vi "Analysis MASTER.vi"(8 "Error In":errorcluster) -> (0 "Error Out":errorcluster)   [LabVIEW 2019, in "MainVIs.lvlib"]
uses:
  MainVIs.lvlib
  Analysis Support/Controls/Select Analysis.ctl
  Analysis Support/Controls/Master Analysis States.ctl
  AnalysisSupport.lvlib
panel:
  out "F0 Array (Mech)":dbl[](array[numeric])
  out "F0 Array (Labial)":dbl[](array[numeric])
  out "SPL Array (Mech)":dbl[](array[numeric])
  out "SPL Array (Labial)":dbl[](array[numeric])
  out "MFR (Labial)":dbl format="%0.3f"
  out "MFR (Mech)":dbl format="%0.3f"
  out "Start Flow (INC)":dbl format="%0.3f"
  out "End Flow (INC)":dbl format="%0.3f"
  out "PTP (INC)":dbl
  out "SPL (INC)":dbl format="%0.3f"
  out "SGP (INC)":dbl
  out "Resistance (INC)":dbl
  out "Pressure (Redirector)":dbl
  out "Filename Out":path
  out "Most Recent File Called":string
  out "SGP Array (Mech)":dbl[](array[numeric])
  out "PTP Array (Mech)":dbl[](array[numeric])
  out "Pressure Array (Labial)":dbl[](array[numeric])
  in  "Begin":bool
  out "Message":string
  in  "Analysis Type":T1 items=["Labial Interruption", "Mechanical Interruption", "Incomplete Interruption", "Airflow Redirection "]
  in  "Exit":bool
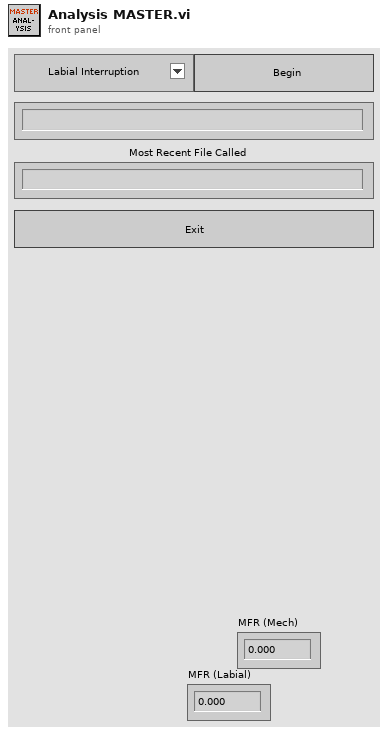
[diagram p1: front panel]
types:
  T1 = typedef "AnalysisSupport.lvlib/Select Analysis.ctl" = u16
  T2 = typedef "AnalysisSupport.lvlib/Master Analysis States.ctl" = enum16{"Initialize", "Wait to Start", "Analyze", "Save", "Timeout", "Exit"}
  T3 = enum16{"Left Button", "Center Button", "Right Button", "Window Close"}
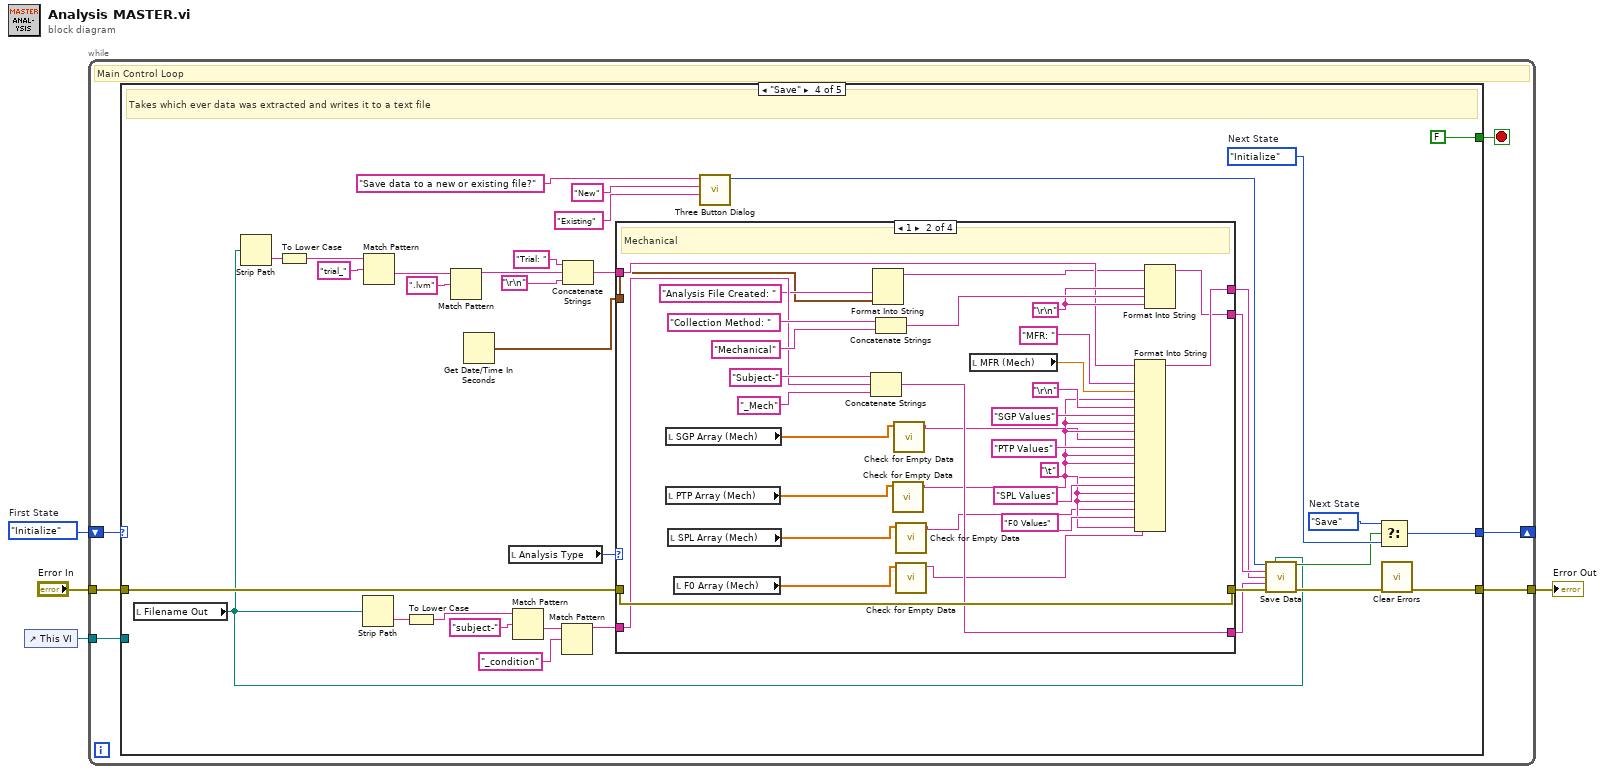
[diagram p0: block diagram]
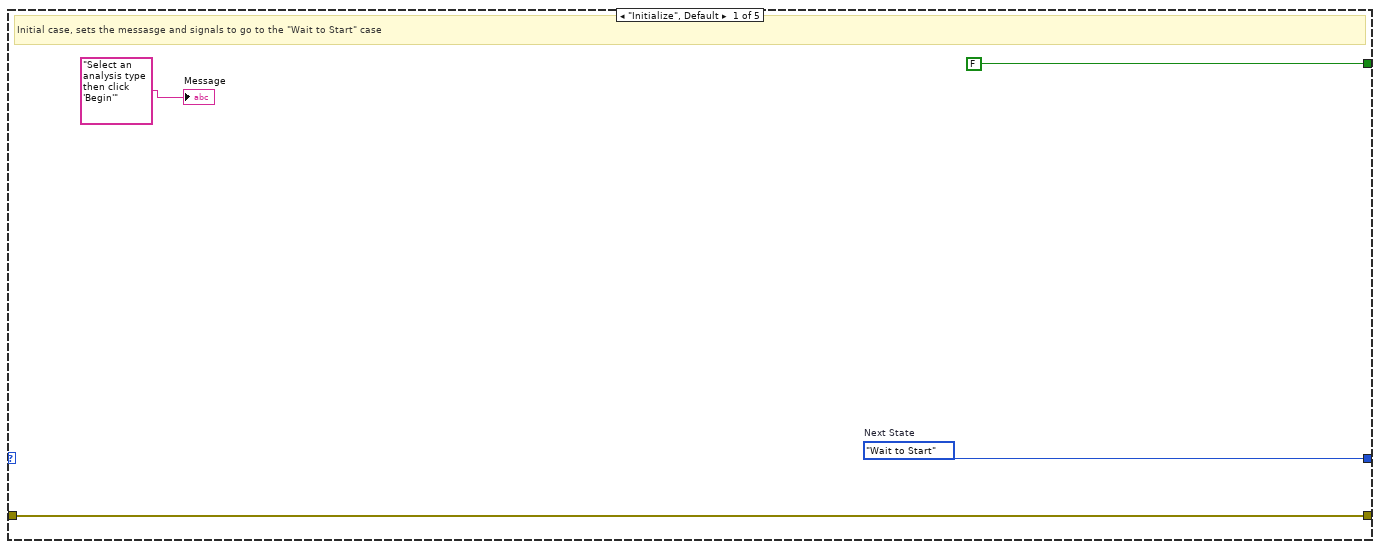
[diagram p2: hidden frame]
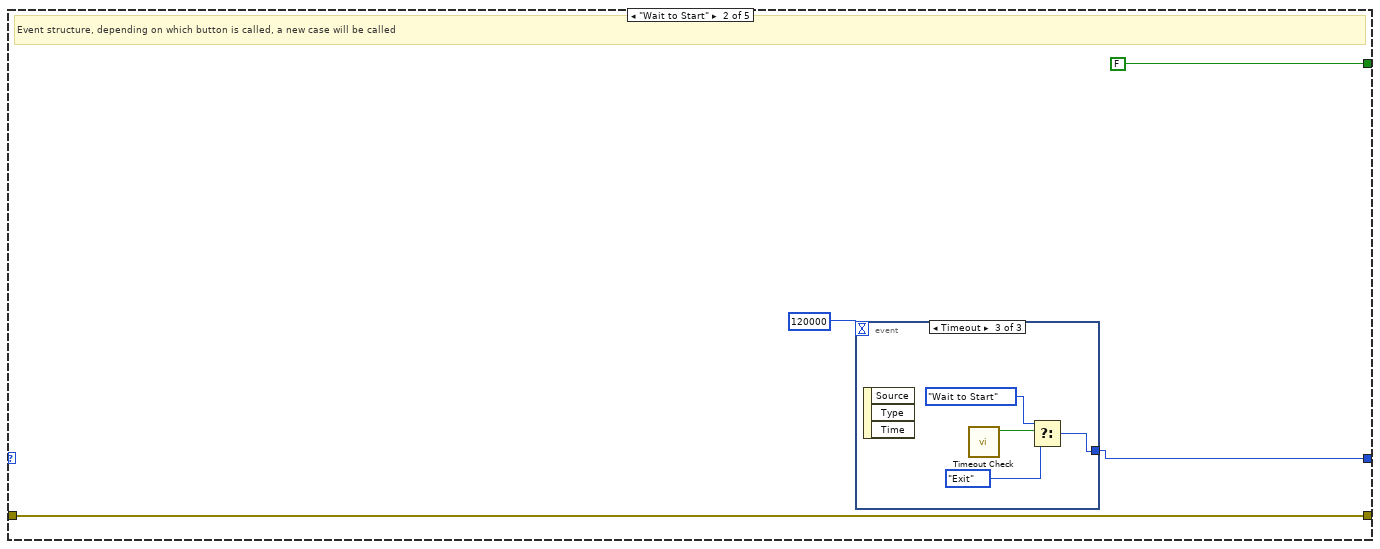
[diagram p3: hidden frame]
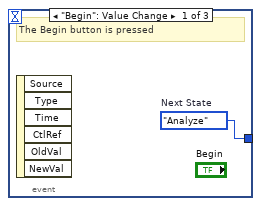
[diagram p4: hidden frame]
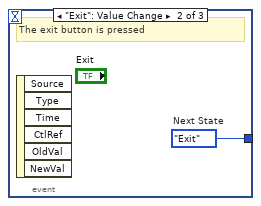
[diagram p5: hidden frame]
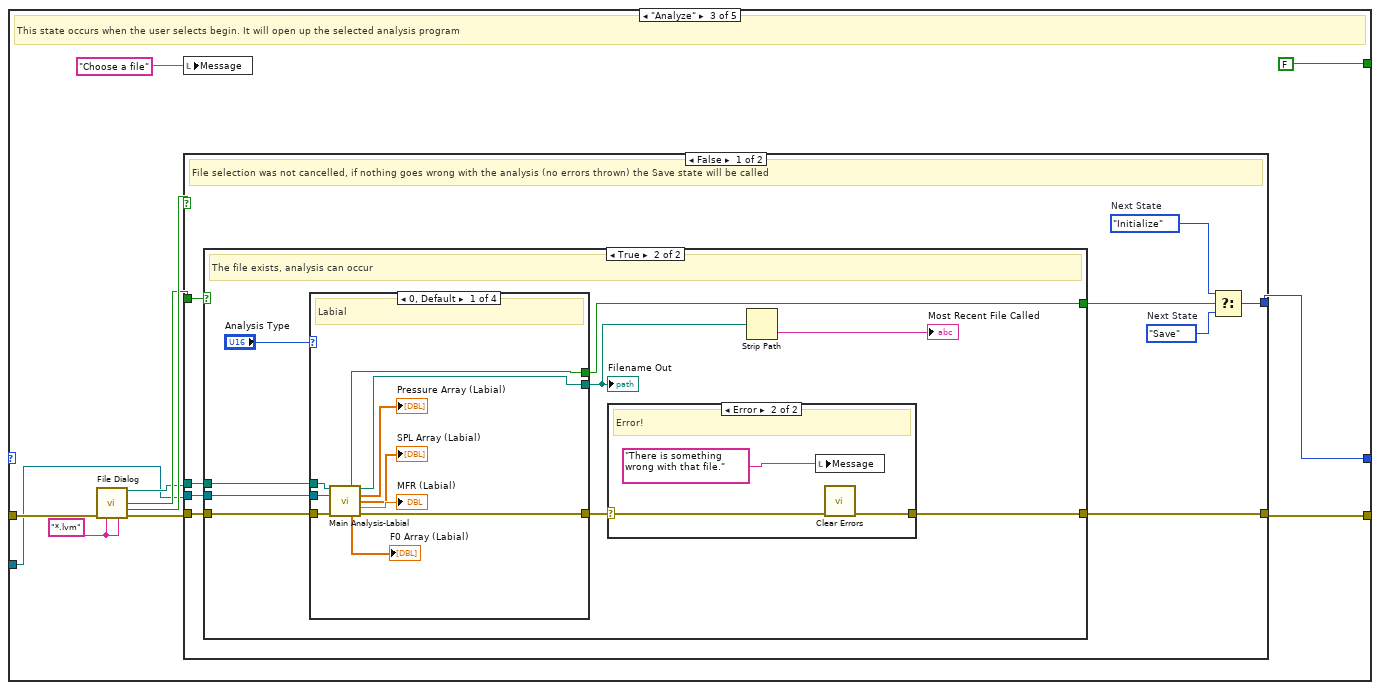
[diagram p6: hidden frame]
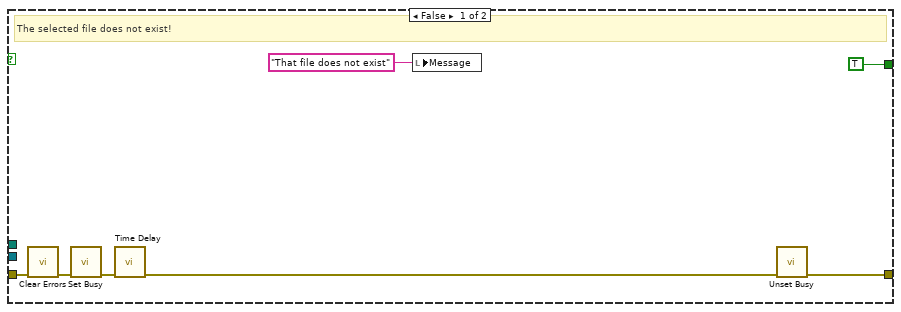
[diagram p7: hidden frame]
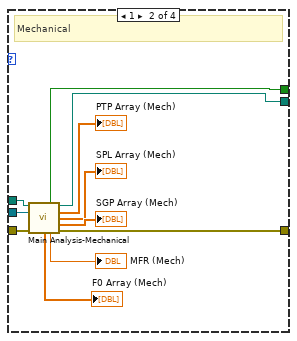
[diagram p9: hidden frame]
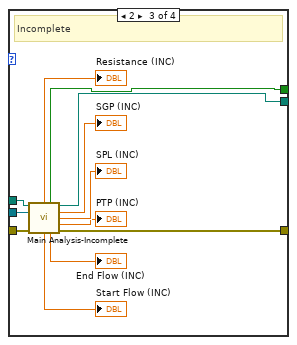
[diagram p10: hidden frame]
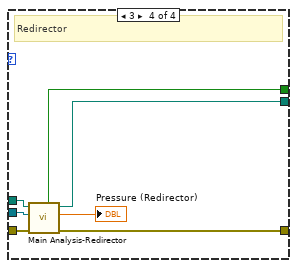
[diagram p11: hidden frame]
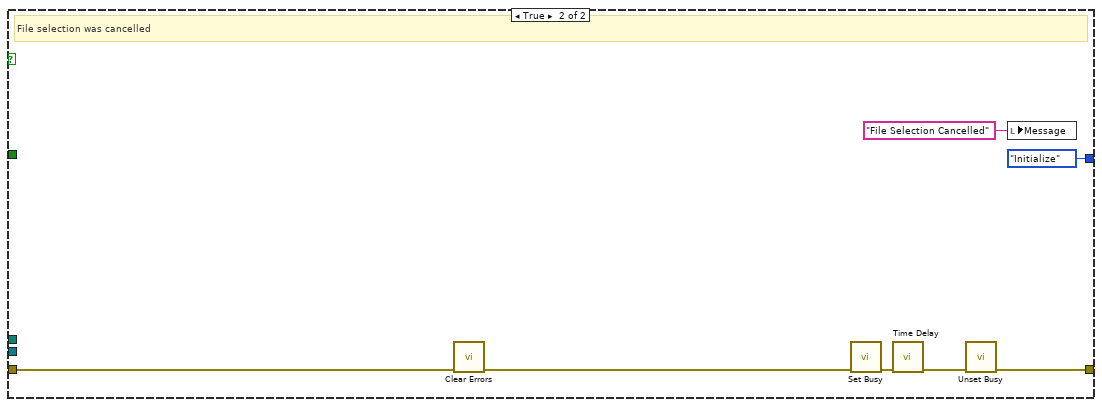
[diagram p12: hidden frame]
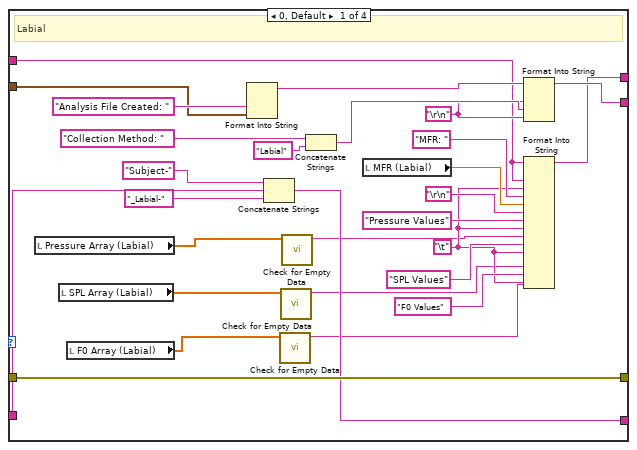
[diagram p13: hidden frame]
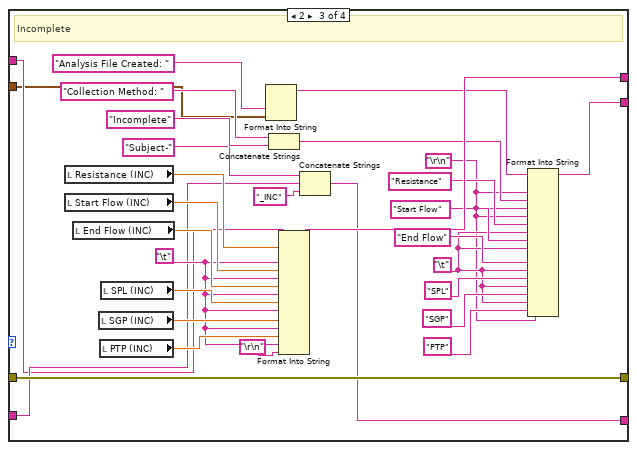
[diagram p14: hidden frame]
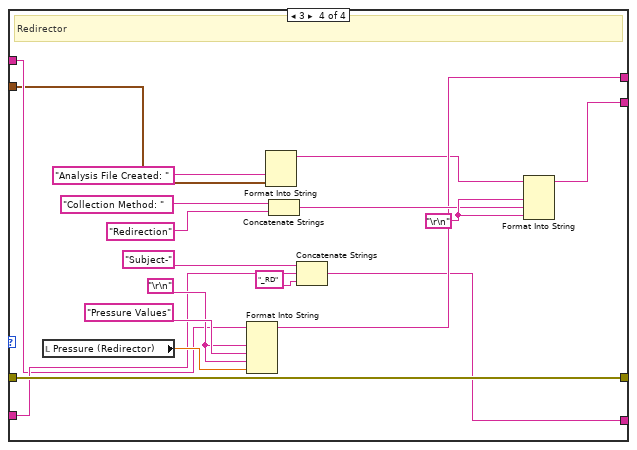
[diagram p15: hidden frame]
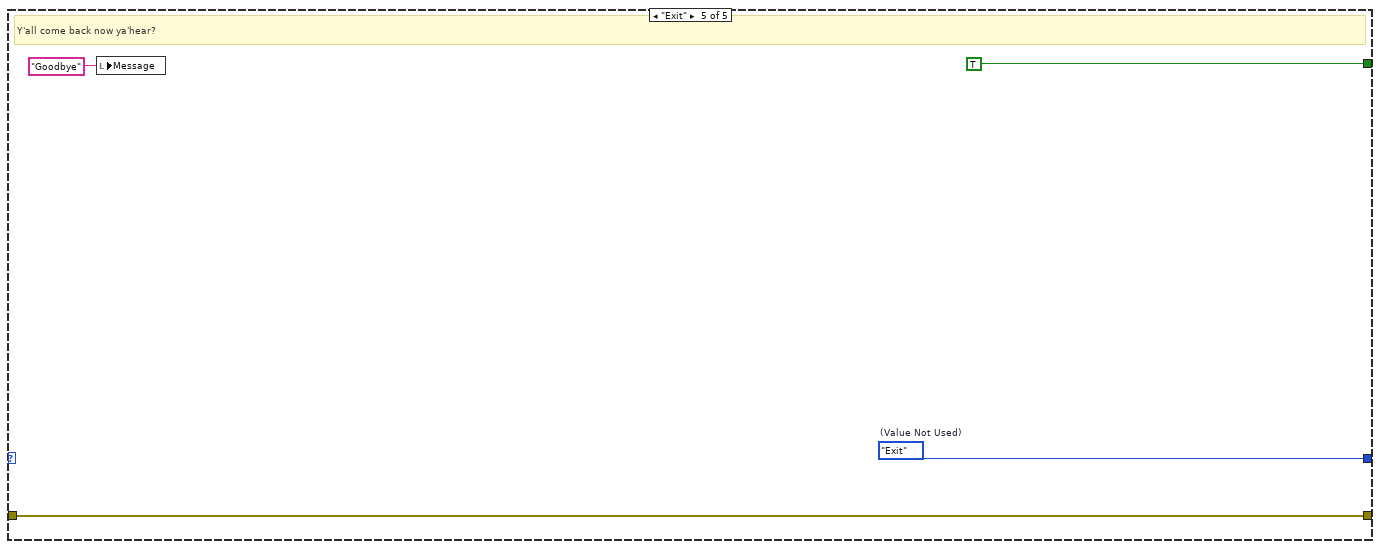
[diagram p16: hidden frame]
diagram:
  w4 = Master_Analysis_States."Initialize"  # First State
  n1 = control-ref of="This VI"() -> (w1:refnum<vi>)
  n2 = while {
    shift-right: [w8] -> _
    shift-left: w4 -> [w10]
    tunnel: "Error In" -> [w7]
    tunnel: [w6] -> w2
    tunnel: w1 -> [w5]
    stop <- w9 stop-if-true
    # "Main Control Loop"
    n3 = case shown="\"Save\"" w10 {
      tunnel: [FALSE FALSE FALSE FALSE TRUE] -> w9
      tunnel: [w12 w18 w26 w122 w255] -> w8
      tunnel: w7 -> [w11 w16 w33 w137 w253]
      tunnel: [w11 w16 w31 w144 w253] -> w6
      tunnel: w5 -> [_ _ w27 _ _]
      frame "Initialize", Default {
        w12 = Master_Analysis_States."Wait to Start"  # Next State
        # "Initial case, sets the messasge and signals to go to the \"Wait to Start\" case"
        "Message" <- "Select an analysis type then click 'Begin'" ("Message")
      }
      frame "Wait to Start" {
        # "Event structure, depending on which button is called, a new case will be called"
        n4 = event shown="[2] Timeout" {
          selector: _ -> [_ _ _]
          dyn-events: _ -> [_ _ _]
          timeout: 120000 -> [_ _ _]
          tunnel: [w19 w20 w21] -> w18
          event "Begin": Value Change {
            w19 = Master_Analysis_States."Analyze"  # Next State
            # "The Begin button is pressed"
            n5 = event-data() -> ()  [unwired: 1 in, 6 out]
          }
          event "Exit": Value Change {
            w20 = Master_Analysis_States."Exit"  # Next State
            # "The exit button is pressed"
            n6 = event-data() -> ()  [unwired: 1 in, 6 out]
          }
          event Timeout {
            n7 = event-data() -> ()  [unwired: 1 in, 3 out]
            n8 = call "Timeout Check.vi"() -> ("Still there?"=w24:bool)  [unwired: 10 in, 1 out]
            n9 = Select(t=Master_Analysis_States."Wait to Start" ("Next State"), s=w24, f=Master_Analysis_States."Exit") -> (s? t:f=w21:T2)
          }
        }
      }
      frame "Analyze" {
        w34 = "*.lvm" ("pattern (all files)")
        # "This state occurs when the user selects begin. It will open up the selected analysis program"
        n10 = call "File Dialog"("error in"=w33, "pattern (all files)"=w34, "pattern label"=w34) -> ("selected path"=w28:path, "exists"=w29:bool, "cancelled"=w30:bool, "error out"=w32:errorcluster)  [unwired: 9 in]
        n11 = local write "Message"("Choose a file" ("Message")) -> ()
        n12 = case shown="False" w30 {
          tunnel: w32 -> [w40 w108]
          tunnel: [w37 w107] -> w31
          tunnel: [w42 Master_Analysis_States."Initialize" ("Next State")] -> w26
          tunnel: w29 -> [w41 _]
          tunnel: w28 -> [w39 _]
          tunnel: w27 -> [w36 _]
          frame False {
            w44 = Master_Analysis_States."Save"  # Next State
            w43 = Master_Analysis_States."Initialize"  # Next State
            # "File selection was not cancelled, if nothing goes wrong with the analysis (no errors thrown) the Save state will be called"
            n13 = case shown="True" w41 {
              tunnel: w40 -> [w47 w60]
              tunnel: [w46 w53] -> w37
              tunnel: w39 -> [_ w57]
              tunnel: [TRUE ("error?") w56] -> w38
              tunnel: w36 -> [_ w52]
              frame False {
                # "The selected file does not exist!"
                n14 = call <vilib>:"Clear Errors.vi"("error in (no error)"=w47) -> ("error out"=w50:errorcluster)  [unwired: 5 in, 1 out]
                n15 = call <vilib>:"Set Busy.vi"("error in (no error)"=w50) -> ("error out"=w48:errorcluster)  [unwired: 9 in, 1 out]
                n16 = call "Time Delay"("error in (no error)"=w48) -> ("error out"=w49:errorcluster)  [unwired: 10 in]
                n17 = local write "Message"("That file does not exist" ("Message")) -> ()
                n18 = call <vilib>:"Unset Busy.vi"("error in (no error)"=w49) -> ("error out"=w46:errorcluster)  [unwired: 10 in]
              }
              frame True {
                # "The file exists, analysis can occur"
                n19 = case shown="0, Default" "Analysis Type" {
                  tunnel: w60 -> [w74 w85 w97 w104]
                  tunnel: [w73 w84 w96 w103] -> w59
                  tunnel: w57 -> [w72 w83 w95 w102]
                  tunnel: [w71 w82 w94 w101] -> w56
                  tunnel: [w70 w81 w93 w100] -> w55
                  tunnel: w52 -> [w66 w76 w86 w98]
                  frame 0, Default {
                    # "Labial"
                    n20 = call "Main Analysis-Labial.vi"("selected path"=w72, "VI reference"=w66, "Error In"=w74) -> ("error?"=w71:bool, "File Path Indicator"=w70:path, "Pressure Array"=→"Pressure Array (Labial)":dbl[], "SPL Array"=→"SPL Array (Labial)":dbl[], "Mean Flow (Overall)"=→"MFR (Labial)":dbl, "F0 Array"=→"F0 Array (Labial)":dbl[], "Error Out"=w73:errorcluster)  [unwired: 6 in]
                  }
                  frame 1 {
                    # "Mechanical"
                    n21 = call "Main Analysis-Mechanical.vi"("selected path"=w83, "VI reference"=w76, "Error In"=w85) -> ("error?"=w82:bool, "Path out"=w81:path, "PTP Array"=→"PTP Array (Mech)":dbl[], "SPL Array"=→"SPL Array (Mech)":dbl[], "SGP Array"=→"SGP Array (Mech)":dbl[], "F0 Array"=→"F0 Array (Mech)":dbl[], "Mean Flow (Overall)"=→"MFR (Mech)":dbl, "Error Out"=w84:errorcluster)  [unwired: 5 in]
                  }
                  frame 2 {
                    # "Incomplete"
                    n22 = call "Main Analysis-Incomplete.vi"("selected path"=w95, "VI reference"=w86, "Error In"=w97) -> ("Resistance (Out)"=→"Resistance (INC)":dbl, "error?"=w94:bool, "Filename Out"=w93:path, "SGP"=→"SGP (INC)":dbl, "SPL"=→"SPL (INC)":dbl, "PTP"=→"PTP (INC)":dbl, "Start Flow"=→"Start Flow (INC)":dbl, "End Flow"=→"End Flow (INC)":dbl, "Error Out"=w96:errorcluster)  [unwired: 4 in]
                  }
                  frame 3 {
                    # "Redirector"
                    n23 = call "Main Analysis-Redirector.vi"("Error In"=w104, "VI reference"=w98, "selected path"=w102) -> ("Error Out"=w103:errorcluster, "Pressure"=→"Pressure (Redirector)":dbl, "Filename Out"=w100:path, "error?"=w101:bool)  [unwired: 5 in]
                  }
                }
                "Filename Out" <- w55
                n24 = case shown="Error" w59 {
                  selector: w59 -> [w61 w63]
                  tunnel: [w61 w62] -> w53
                  frame No Error {
                    # "No Errors! YAY!"
                  }
                  frame Error {
                    # "Error!"
                    n25 = local write "Message"("There is something wrong with that file." ("Message")) -> ()
                    n26 = call <vilib>:"Clear Errors.vi"("error in (no error)"=w63) -> ("error out"=w62:errorcluster)  [unwired: 5 in, 1 out]
                  }
                }
                n27 = Strip Path(path=w55) -> (name=→"Most Recent File Called":string)  [unwired: 1 out]
              }
            }
            n28 = Select(t=w43, s=w38, f=w44) -> (s? t:f=w42:T2)
          }
          frame True {
            # "File selection was cancelled"
            n29 = call <vilib>:"Clear Errors.vi"("error in (no error)"=w108) -> ("error out"=w110:errorcluster)  [unwired: 5 in, 1 out]
            n30 = call <vilib>:"Set Busy.vi"("error in (no error)"=w110) -> ("error out"=w109:errorcluster)  [unwired: 9 in, 1 out]
            n31 = call "Time Delay"("error in (no error)"=w109) -> ("error out"=w111:errorcluster)  [unwired: 10 in]
            n32 = call <vilib>:"Unset Busy.vi"("error in (no error)"=w111) -> ("error out"=w107:errorcluster)  [unwired: 10 in]
            n33 = local write "Message"("File Selection Cancelled" ("Message")) -> ()
          }
        }
      }
      frame "Save" {
        w125 = Master_Analysis_States."Save"  # Next State
        w124 = Master_Analysis_States."Initialize"  # Next State
        # "Takes which ever data was extracted and writes it to a text file"
        n34 = local read "Filename Out"() -> (w120:path)
        n35 = Strip Path(path=w120) -> (name=w121:string)  [unwired: 1 out]
        n36 = To Lower Case(string=w121) -> (all lower case string=w119:string)
        n37 = Strip Path(path=w120) -> (name=w126:string)  [unwired: 1 out]
        n38 = Match Pattern(string=w119, regular expression="trial_") -> (after substring=w114:string)  [unwired: 1 in, 3 out]
        n39 = To Lower Case(string=w126) -> (all lower case string=w127:string)
        n40 = Match Pattern(string=w114, regular expression=".lvm") -> (before substring=w112:string)  [unwired: 1 in, 3 out]
        n41 = Get Date/Time In Seconds() -> (seconds since 1Jan1904=w133:timestamp)
        n42 = local read "Analysis Type"() -> (w138:T1)
        n43 = Match Pattern(string=w127, regular expression="subject-") -> (after substring=w128:string)  [unwired: 1 in, 3 out]
        n44 = Match Pattern(string=w128, regular expression="_condition") -> (before substring=w129:string)  [unwired: 1 in, 3 out]
        n45 = Concatenate Strings("Trial: " ("string"), w112, "\r\n") -> (w115:string)
        n46 = case shown="1" w138 {
          tunnel: w137 -> [w169 w201 w234 w252]
          tunnel: [w169 w201 w234 w252] -> w136
          tunnel: [w171 w200 w229 w247] -> w135
          tunnel: [w170 w202 w231 w245] -> w134
          tunnel: w133 -> [w158 w187 w206 w236]
          tunnel: [w163 w191 w209 w239] -> w131
          tunnel: w129 -> [w165 w193 w211 w241]
          tunnel: w115 -> [w155 w189 w208 w238]
          frame 0, Default {
            w152 = "\t"
            w167 = "\r\n"
            # "Labial"
            n47 = local read "Pressure Array (Labial)"() -> (w147:dbl[])
            n48 = local read "SPL Array (Labial)"() -> (w149:dbl[])
            n49 = local read "F0 Array (Labial)"() -> (w150:dbl[])
            n50 = Format Into String "Format Into String"("Analysis File Created: ", w158) -> (resulting string=w157:string)  [unwired: 3 in, 1 out]
            n51 = Concatenate Strings("Subject-" ("string"), w165, "_Labial-" ("string")) -> (w163:string)
            n52 = call "Check for Empty Data.vi"("F0 Array (Labial)"=w150) -> ("spreadsheet string"=w151:string)  [unwired: 10 in]
            n53 = call "Check for Empty Data.vi"("F0 Array (Labial)"=w149) -> ("spreadsheet string"=w148:string)  [unwired: 10 in]
            n54 = call "Check for Empty Data.vi"("F0 Array (Labial)"=w147) -> ("spreadsheet string"=w146:string)  [unwired: 10 in]
            n55 = Concatenate Strings("Collection Method: ", "Labial" ("string")) -> (w168:string)
            n56 = local read "MFR (Labial)"() -> (w161:dbl)
            n57 = Format Into String "Format Into String"(initial string=w157, w167, w168, w167) -> (resulting string=w171:string)  [unwired: 2 in, 1 out]
            n58 = Format Into String "Format Into String"(initial string=w155, w155, w152, "MFR: ", w161, "\r\n", "Pressure Values" ("input 2"), w152, w146, "SPL Values" ("input 6"), w152, w148, "F0 Values" ("input 12"), w152, w151) -> (resulting string=w170:string)  [unwired: 2 in, 1 out]
          }
          frame 1 {
            w182 = "\t"
            w198 = "\r\n"
            # "Mechanical"
            n59 = local read "SGP Array (Mech)"() -> (w181:dbl[])
            n60 = local read "PTP Array (Mech)"() -> (w176:dbl[])
            n61 = local read "SPL Array (Mech)"() -> (w175:dbl[])
            n62 = local read "F0 Array (Mech)"() -> (w179:dbl[])
            n63 = Concatenate Strings("Subject-" ("default name"), w193, "_Mech" ("string")) -> (w191:string)
            n64 = Format Into String("Analysis File Created: ", w187) -> (resulting string=w186:string)  [unwired: 3 in, 1 out]
            n65 = Concatenate Strings("Collection Method: ", "Mechanical") -> (w199:string)
            n66 = call "Check for Empty Data.vi"("F0 Array (Labial)"=w176) -> ("spreadsheet string"=w177:string)  [unwired: 10 in]
            n67 = call "Check for Empty Data.vi"("F0 Array (Labial)"=w181) -> ("spreadsheet string"=w180:string)  [unwired: 10 in]
            n68 = call "Check for Empty Data.vi"("F0 Array (Labial)"=w175) -> ("spreadsheet string"=w174:string)  [unwired: 10 in]
            n69 = call "Check for Empty Data.vi"("F0 Array (Labial)"=w179) -> ("spreadsheet string"=w178:string)  [unwired: 10 in]
            n70 = local read "MFR (Mech)"() -> (w184:dbl)
            n71 = Format Into String(initial string=w189, "MFR: ", w184, w182, "\r\n", "SGP Values" ("input 1"), w182, w182, w180, "PTP Values" ("input 6"), w182, w182, w177, "SPL Values" ("input 6"), w182, w182, w174, "F0 Values" ("input 17"), w182, w178) -> (resulting string=w202:string)  [unwired: 2 in, 1 out]
            n72 = Format Into String(initial string=w186, w198, w199, w198) -> (resulting string=w200:string)  [unwired: 2 in, 1 out]
          }
          frame 2 {
            w218 = "\t"
            w214 = "\t"
            w216 = "\r\n"
            # "Incomplete"
            n73 = local read "Resistance (INC)"() -> (w228:dbl)
            n74 = local read "Start Flow (INC)"() -> (w226:dbl)
            n75 = local read "End Flow (INC)"() -> (w224:dbl)
            n76 = local read "SGP (INC)"() -> (w220:dbl)
            n77 = local read "PTP (INC)"() -> (w215:dbl)
            n78 = local read "SPL (INC)"() -> (w222:dbl)
            n79 = Format Into String("Analysis File Created: ", w206) -> (resulting string=w205:string)  [unwired: 3 in, 1 out]
            n80 = Concatenate Strings("Collection Method: ", "Incomplete") -> (w230:string)
            n81 = Format Into String(initial string=w208, w228, w214, w226, w214, w224, w214, w222, w214, w220, w214, w215, w214, "\r\n") -> (resulting string=w231:string)  [unwired: 2 in, 1 out]
            n82 = Concatenate Strings("Subject-" ("default name"), w211, "_INC" ("string")) -> (w209:string)
            n83 = Format Into String(initial string=w205, w216, w230, w216, w216, "Resistance" ("input 7"), w218, "Start Flow" ("input 9"), w218, "End Flow" ("input 11"), w218, "SPL" ("input 13"), w218, "SGP" ("input 15"), w218, "PTP" ("input 17"), w216) -> (resulting string=w229:string)  [unwired: 2 in, 1 out]
          }
          frame 3 {
            w244 = "\r\n"
            w249 = "\r\n"
            # "Redirector"
            n84 = local read "Pressure (Redirector)"() -> (w243:dbl)
            n85 = Format Into String "Format Into String"(initial string=w238, w244, "Pressure Values" ("input 2"), w244, w243) -> (resulting string=w245:string)  [unwired: 2 in, 1 out]
            n86 = Format Into String("Analysis File Created: ", w236) -> (resulting string=w235:string)  [unwired: 3 in, 1 out]
            n87 = Concatenate Strings("Collection Method: ", "Redirection" ("string")) -> (w248:string)
            n88 = Concatenate Strings("Subject-" ("default name"), w241, "_RD" ("string")) -> (w239:string)
            n89 = Format Into String "Format Into String"(initial string=w235, w249, w248, w249) -> (resulting string=w247:string)  [unwired: 2 in, 1 out]
          }
        }
        n90 = call <vilib>:"Three Button Dialog.vi"("Center Button Text (\"No\")"="Existing" ("T button name (\"OK\")"), "Left Button Text (\"Yes\")"="New" ("F button name (\"Cancel\")"), "message"="Save data to a new or existing file?") -> ("Which Button?"=w139:T3)  [unwired: 8 in]
        n91 = call "Save Data.vi"("Which Button?"=w139, "start path"=w120, "Header (If NEW is selected)"=w135, "Data to be saved (String)"=w134, "default name"=w131, "error in (no error)"=w136) -> ("Maybe go back?"=w123:bool, "error out"=w143:errorcluster)  [unwired: 8 in]
        n92 = Select(t=w125, s=w123, f=w124) -> (s? t:f=w122:T2)
        n93 = call <vilib>:"Clear Errors.vi"("error in (no error)"=w143) -> ("error out"=w144:errorcluster)  [unwired: 5 in, 1 out]
      }
      frame "Exit" {
        w255 = Master_Analysis_States."Exit"  # (Value Not Used)
        # "Y'all come back now ya'hear?"
        n94 = local write "Message"("Goodbye" ("Message")) -> ()
      }
    }
  }
  "Error Out" <- w2
